vi "SVFA Get Spectrum Subset.vi"   [LabVIEW 2017]
doc: "Extracts the subset of the spectrum specified by <B>range</B>. <B>x0</B> is updated to reflect the new start frequency, <B>dx</B> is the same as in the input spectrum, and the spectrum array is shortened so the last element corresponds with the stop value specified in the <B>range</B>. Use this VI for operations such as limiting subsequent spectrum operations to the region of interest or removing the part of the spectrum outside the alias-free bandwidth, as well as others. Wire data to the <B>spectrum</B> input to determine the polymorphic instance to use or manually select the instance."
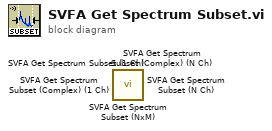
[diagram p0: block diagram]
diagram:
  n1 = call <vilib>:"SVFA Get Spectrum Subset (NxM).vi"() -> ()  [unwired: 14 in, 6 out]
  n2 = call <vilib>:"SVFA Get Spectrum Subset (Complex) (N Ch).vi"() -> ()  [unwired: 16 in, 4 out]
  n3 = call <vilib>:"SVFA Get Spectrum Subset (Complex) (1 Ch).vi"() -> ()  [unwired: 16 in, 4 out]
  n4 = call <vilib>:"SVFA Get Spectrum Subset (N Ch).vi"() -> ()  [unwired: 14 in, 6 out]
  n5 = call <vilib>:"SVFA Get Spectrum Subset (1 Ch).vi"() -> ()  [unwired: 14 in, 6 out]
